vi "Initialized.vi"(8 "error in":errorcluster) -> (0 "error out":errorcluster, 2 "Initialized?":bool)   [LabVIEW 2019, in "Identifier.lvclass"]
uses:
  Identifier.lvclass
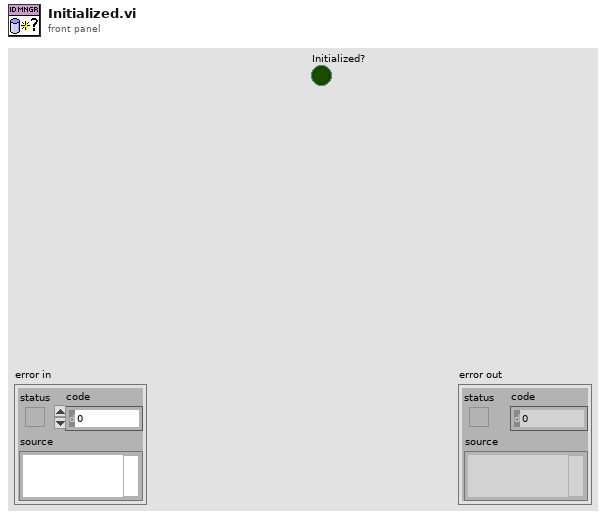
[diagram p1: front panel]
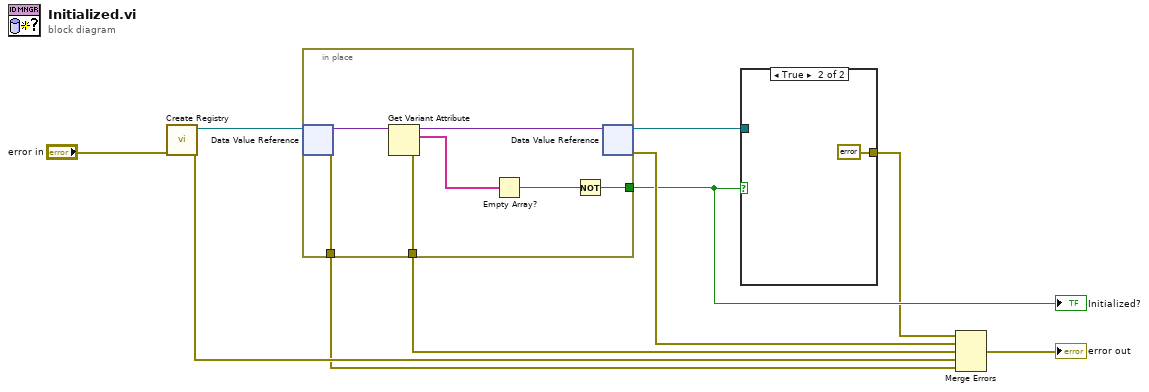
[diagram p0: block diagram]
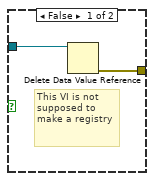
[diagram p2: hidden frame]
diagram:
  n1 = call "Create Registry.vi"("error in"="error in") -> ("error out"=w8:errorcluster, "Registry"=w9:refnum<data-value>)  [unwired: 9 in]
  n2 = in-place {
    in-place-border: [w13] -> w3
    in-place-border: [w12] -> w7
    in-place-border: [w11] -> w6
    n3 = in-place-dvr #1(w9) -> (w17:variant, w12:errorcluster)
    n4 = Get Variant Attribute(Variant=w17) -> (duplicate Variant=w16:variant, names=w15:string[], error out=w11:errorcluster)  [unwired: 3 in, 1 out]
    n5 = Empty Array?(array=w15) -> (empty?=w14:bool)
    n6 = Not(x=w14) -> (.not. x?=w13:bool)
    n7 = in-place-dvr #1(w16) -> (w2:refnum<data-value>, w5:errorcluster)
  }
  "Initialized?" <- w3
  n8 = case shown="True" w3 {
    tunnel: w2 -> [w19 _]
    tunnel: [w18 errorcluster {"status"=FALSE, "code"=0, "source"=""} ("error out")] -> w1
    frame False {
      # "This VI is not supposed to make a registry"
      n9 = Delete Data Value Reference(data value reference=w19) -> (error out=w18:errorcluster)  [unwired: 1 in, 1 out]
    }
    frame True {
    }
  }
  n10 = Merge Errors(w1, w5, w6, w8, w7) -> (→"error out":errorcluster)
